vi "MOCVD_FrontPanel.vi"() -> ()   [LabVIEW 2011]
uses:
  low_level_proc/globals.vi
  editor_lib/Flow_Globals.vi
panel:
  out "Temp Actual":dbl caption="Actual (C)" format="%.2f"
  in  "Set":bool
  in  "Temp Setpoint":dbl caption="Setpoint (C)"
  in  "Heater":bool
  in  "Spinner":bool
  in  "Heater/Spinner Remote":bool caption="Remote"
  in  "Vac Remote":bool
  in  "Vac Exhaust":bool
  in  "Atm Exhaust":bool
  in  "Clear All Relays":bool
  in  "Stop":bool
  in  "?":enum32{"N2/H2", "Al", "Ga", "In", "P", "As"}(tab)
  in  "display N2 or H2":bool=TRUE
  in  "H2N2 Remote":bool caption="Remote"
  in  "N2 Target Flow":dbl caption="Target" min=0.0 max=1000.0
  in  "H2 Target Flow":dbl caption="Target" min=0.0 max=1000.0
  out "H2N2 Actual Flow":dbl caption="Actual"
  in  "N2 On":bool caption="On"
  in  "H2 On":bool caption="On"
  in  "Al Target Flow":dbl caption="Target" min=0.0 max=100.0 format="%.1f"
  out "Al Actual Flow":dbl caption="Actual" format="%.1f"
  in  "Al Remote":bool caption="Remote"
  in  "Al Active":bool caption="Active"
  in  "Al Bubbler In":bool caption="Bubbler In"
  in  "Al Run":bool caption="Run"
  out "Ga Actual Flow2":dbl caption="Actual" format="%.2f"
  out "Ga Actual Flow1":dbl caption="Actual" format="%.2f"
  out "Ga Actual Flow3":dbl caption="Actual"
  in  "Ga Target Flow 2":dbl caption="Target" min=0.0 max=10.0 format="%.2f"
  in  "Ga Target Flow 1":dbl caption="Target" min=0.0 max=1.0 format="%.2f"
  in  "Ga Active":bool caption="Active"
  in  "Ga Bubbler In":bool caption="Bubbler In"
  in  "Ga Run":bool caption="Run"
  in  "Ga H2 Dilute":bool caption="H2 Dilute"
  in  "Ga Remote":bool caption="Remote"
  in  "Ga Target Flow 3":dbl caption="Target" min=0.0 max=1000.0
  in  "In Target Flow":dbl caption="Target" min=0.0 max=100.0 format="%.1f"
  out "In Actual Flow":dbl caption="Actual" format="%.1f"
  in  "In Remote":bool caption="Remote"
  in  "In Active":bool caption="Active"
  in  "In Bubbler In":bool caption="Bubbler In"
  in  "In Run":bool caption="Run"
  in  "P_gas Target Flow":dbl caption="Target" min=0.0 max=1000.0 format="%.1f"
  out "P Actual Flow":dbl caption="Actual" format="%.1f"
  in  "P gas Remote":bool caption="Remote"
  in  "P gas Active":bool caption="Active"
  in  "P Gas In":bool caption="Gas In"
  in  "P gas Run":bool caption="Run"
  in  "P gas H2 Purge":bool caption="H2 Purge"
  in  "AsH3 gas Target Flow":dbl caption="Target" min=0.0 max=1000.0 format="%.2f"
  out "As Actual Flow":dbl caption="Actual" format="%.2f"
  in  "As gas Run":bool caption="Run"
  in  "As gas H2 Purge":bool caption="H2 Purge"
  in  "As gas Active":bool caption="Active"
  in  "As Gas In":bool caption="Gas In"
  in  "As gas Remote":bool caption="Remote"
  in  "6940B GPIB Address":string="23"
  # "Flow (0-10000 sccm)"
  # "N2"
  # "H2"
  # "N2"
  # "H2"
  # "Flow (0-100 sscm)"
  # "Flow 1 (0-10 sscm)"
  # "Flow 2 (0-10 sscm)"
  # "Flow 3 (0-1000 sscm)"
  # "Flow (0-100 sscm)"
  # "Flow (0-100 sscm)"
  # "Flow (0-10 sscm)"
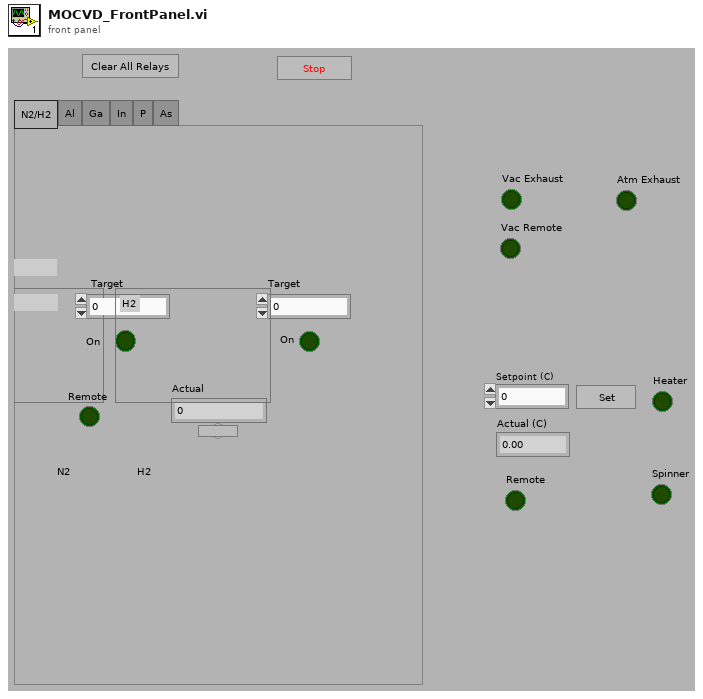
[diagram p1: front panel]
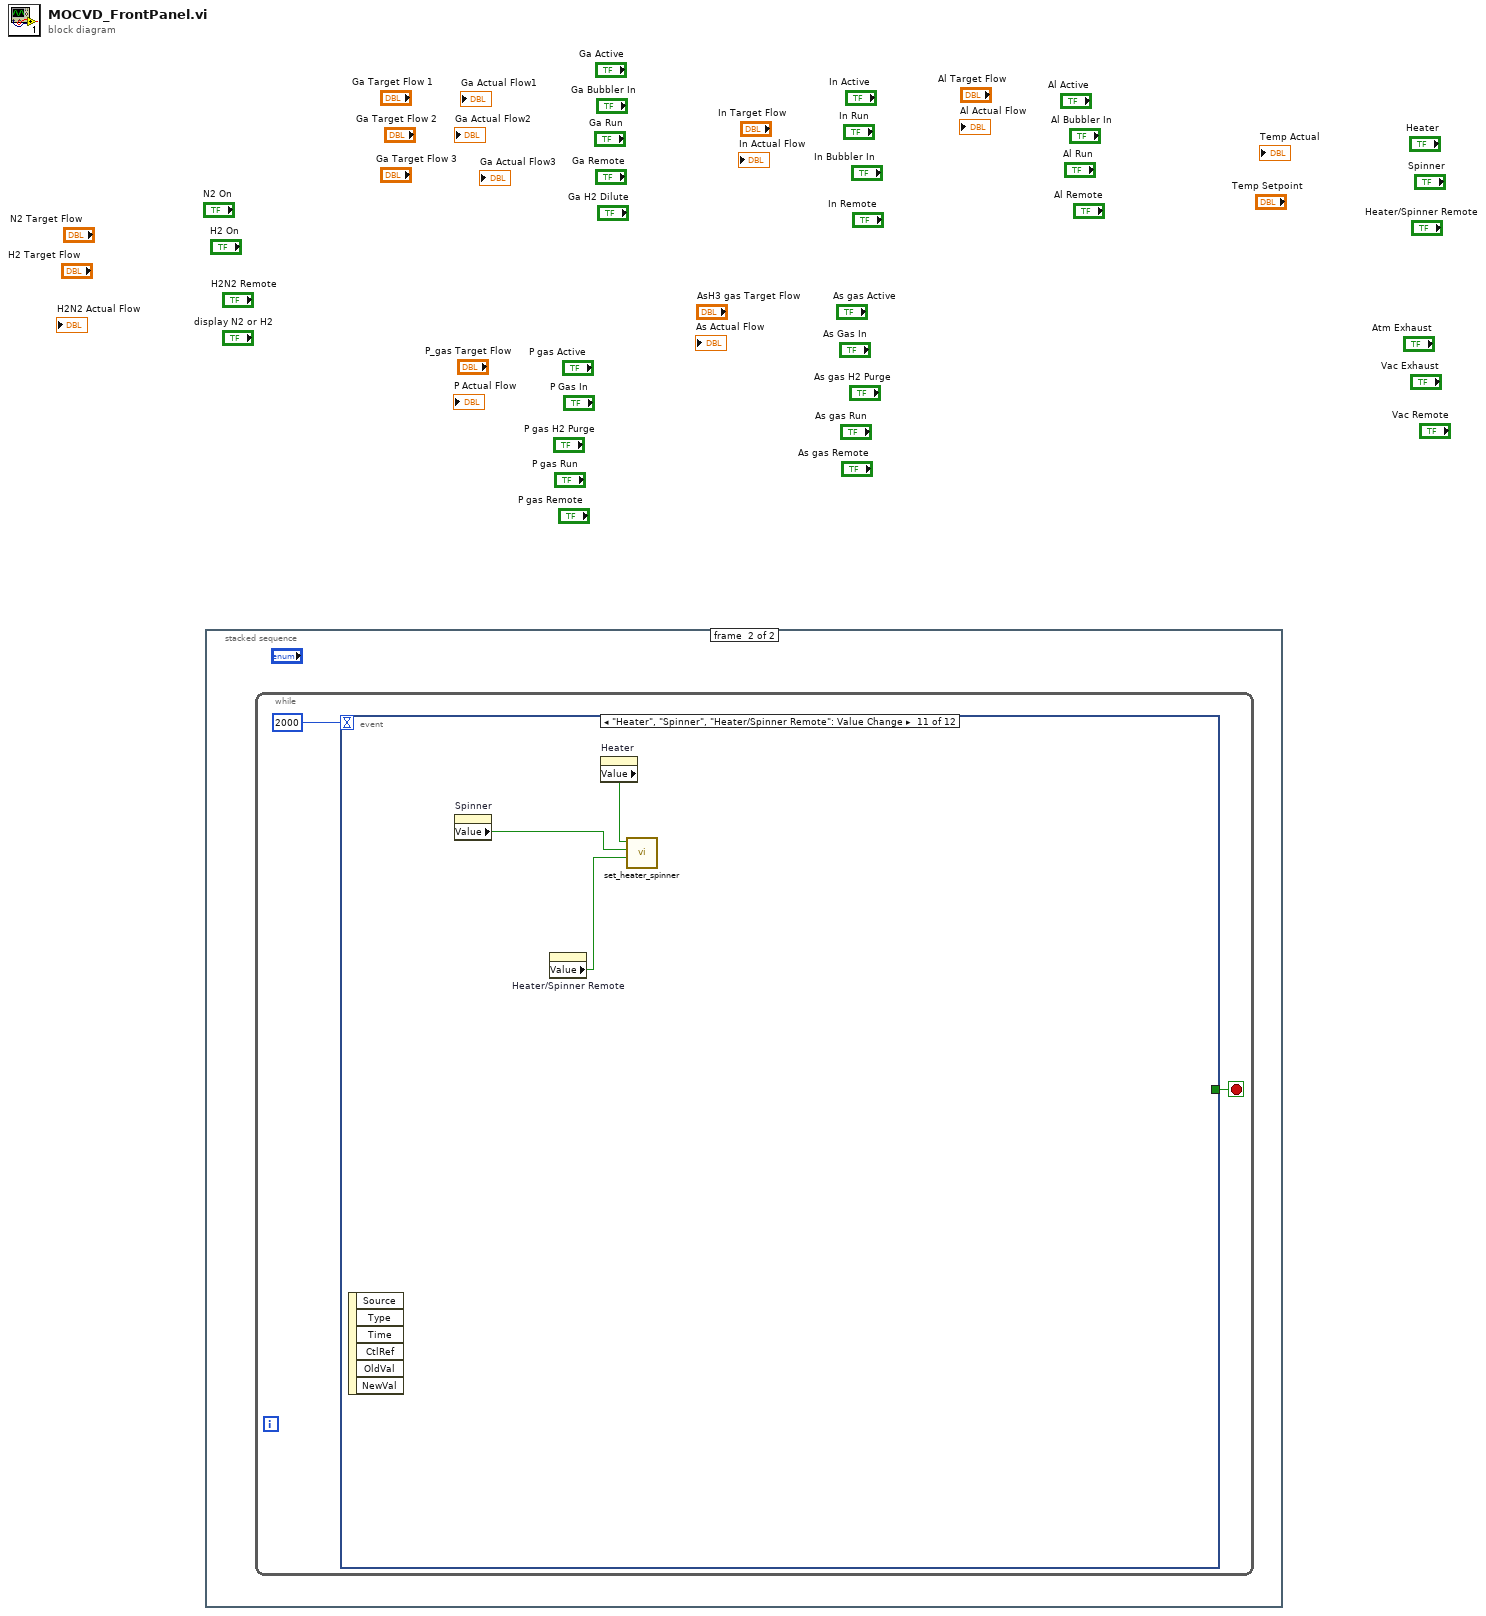
[diagram p0: block diagram]
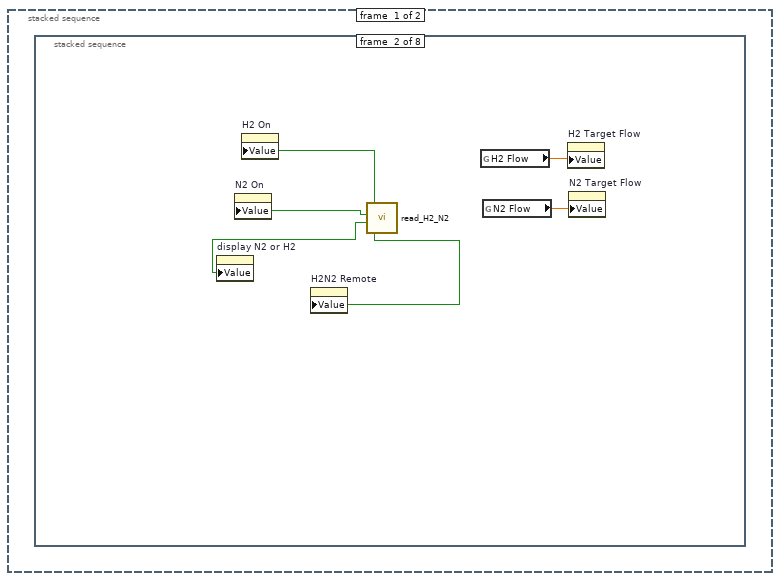
[diagram p2: hidden frame]
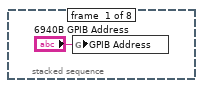
[diagram p3: hidden frame]
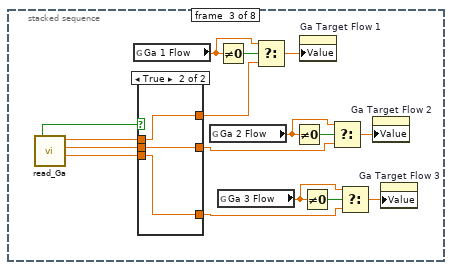
[diagram p4: hidden frame]
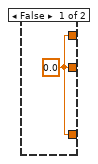
[diagram p5: hidden frame]
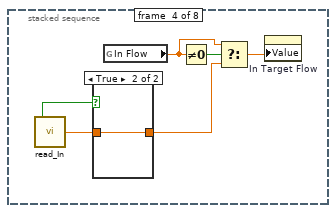
[diagram p6: hidden frame]
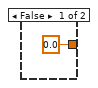
[diagram p7: hidden frame]
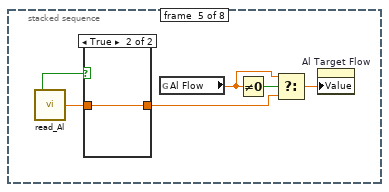
[diagram p8: hidden frame]
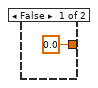
[diagram p9: hidden frame]
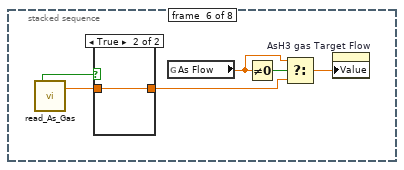
[diagram p10: hidden frame]
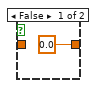
[diagram p11: hidden frame]
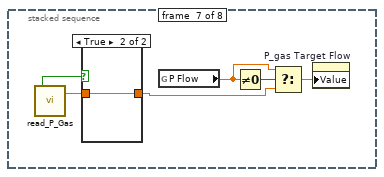
[diagram p12: hidden frame]
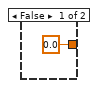
[diagram p13: hidden frame]
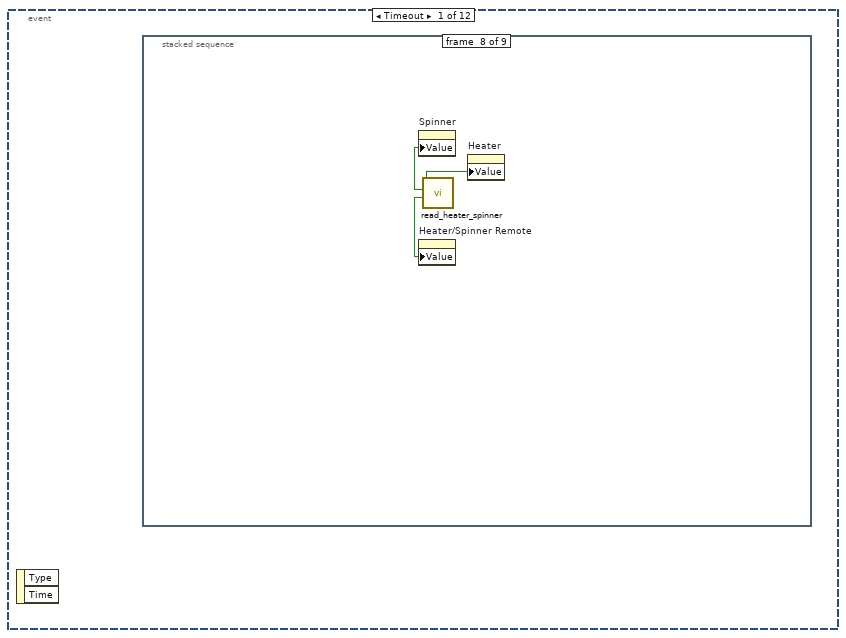
[diagram p15: hidden frame]
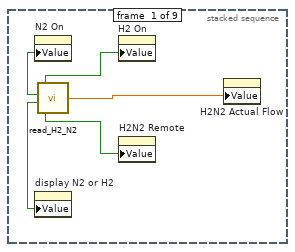
[diagram p16: hidden frame]
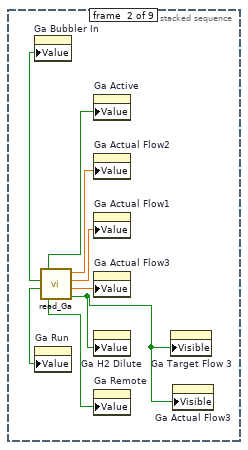
[diagram p17: hidden frame]
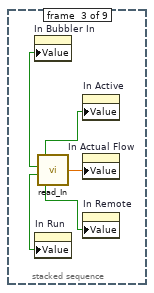
[diagram p18: hidden frame]
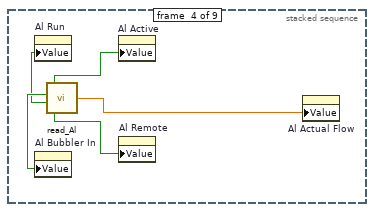
[diagram p19: hidden frame]
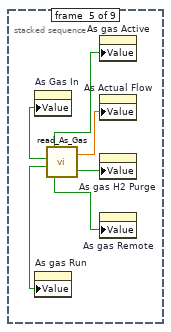
[diagram p20: hidden frame]
diagram:
  n1 = stacked-sequence {
    frame #0 {
      n2 = stacked-sequence {
        frame #0 {
          n3 = global write "globals.vi" "GPIB Address"("6940B GPIB Address") -> ()
        }
        frame #1 {
          n4 = call "read_H2_N2.vi"() -> ("H2N2 Remote"=w5:bool, "Display H2N2"=w4:bool, "N2 Active"=w7:bool, "H2 Active"=w6:bool)  [unwired: 1 out]
          n5 = property on="display N2 or H2" class="Bool (strict)"("Value"=w4) -> ()  [unwired: 2 in, 2 out]
          n6 = property on="N2 On" class="Bool (strict)"("Value"=w7) -> ()  [unwired: 2 in, 2 out]
          n7 = property on="H2 On" class="Bool (strict)"("Value"=w6) -> ()  [unwired: 2 in, 2 out]
          n8 = property on="H2N2 Remote" class="Bool (strict)"("Value"=w5) -> ()  [unwired: 2 in, 2 out]
          n9 = global read "Flow_Globals.vi" "H2 Flow"() -> (w3:dbl)
          n10 = global read "Flow_Globals.vi" "N2 Flow"() -> (w2:dbl)
          n11 = property on="H2 Target Flow" class="DigNum (strict)"("Value"=w3) -> ()  [unwired: 2 in, 2 out]
          n12 = property on="N2 Target Flow" class="DigNum (strict)"("Value"=w2) -> ()  [unwired: 2 in, 2 out]
        }
        frame #2 {
          n13 = call "read_Ga.vi"() -> ("GAMFC3"=w22:dbl, "GAMFC2"=w23:dbl, "GAMFC1"=w21:dbl, "Ga Active"=w20:bool)  [unwired: 4 out]
          n14 = global read "Flow_Globals.vi" "Ga 1 Flow"() -> (w18:dbl)
          n15 = case shown="True" w20 {
            tunnel: w23 -> [_ w26]
            tunnel: w22 -> [_ w25]
            tunnel: w21 -> [_ w27]
            tunnel: [w24 w27] -> w17
            tunnel: [w24 w26] -> w13
            tunnel: [w24 w25] -> w9
            frame False {
              w24 = 0.0 ("GAMFC2")
            }
            frame True {
            }
          }
          n16 = global read "Flow_Globals.vi" "Ga 2 Flow"() -> (w14:dbl)
          n17 = Not Equal To 0?(x=w18) -> (x != 0?=w19:bool)
          n18 = global read "Flow_Globals.vi" "Ga 3 Flow"() -> (w10:dbl)
          n19 = Select(t=w18, s=w19, f=w17) -> (s? t:f=w16:dbl)
          n20 = Not Equal To 0?(x=w14) -> (x != 0?=w15:bool)
          n21 = property on="Ga Target Flow 1" class="DigNum (strict)"("Value"=w16) -> ()  [unwired: 2 in, 2 out]
          n22 = Not Equal To 0?(x=w10) -> (x != 0?=w11:bool)
          n23 = Select(t=w14, s=w15, f=w13) -> (s? t:f=w12:dbl)
          n24 = Select(t=w10, s=w11, f=w9) -> (s? t:f=w8:dbl)
          n25 = property on="Ga Target Flow 2" class="DigNum (strict)"("Value"=w12) -> ()  [unwired: 2 in, 2 out]
          n26 = property on="Ga Target Flow 3" class="DigNum (strict)"("Value"=w8) -> ()  [unwired: 2 in, 2 out]
        }
        frame #3 {
          n27 = call "read_In.vi"() -> ("Actual In Flow Rate"=w32:dbl, "In Active"=w33:bool)  [unwired: 3 out]
          n28 = case shown="True" w33 {
            tunnel: [0.0 ("Actual In Flow Rate") w35] -> w29
            tunnel: w32 -> [_ w35]
            frame False {
            }
            frame True {
            }
          }
          n29 = global read "Flow_Globals.vi" "In Flow"() -> (w30:dbl)
          n30 = Not Equal To 0?(x=w30) -> (x != 0?=w31:bool)
          n31 = Select(t=w30, s=w31, f=w29) -> (s? t:f=w28:dbl)
          n32 = property on="In Target Flow" class="DigNum (strict)"("Value"=w28) -> ()  [unwired: 2 in, 2 out]
        }
        frame #4 {
          n33 = call "read_Al.vi"() -> ("Actual Al Flow Rate"=w41:dbl, "Al Active"=w40:bool)  [unwired: 3 out]
          n34 = case shown="True" w40 {
            tunnel: [0.0 ("Actual Al Flow Rate") w43] -> w37
            tunnel: w41 -> [_ w43]
            frame False {
            }
            frame True {
            }
          }
          n35 = global read "Flow_Globals.vi" "Al Flow"() -> (w38:dbl)
          n36 = Not Equal To 0?(x=w38) -> (x != 0?=w39:bool)
          n37 = Select(t=w38, s=w39, f=w37) -> (s? t:f=w36:dbl)
          n38 = property on="Al Target Flow" class="DigNum (strict)"("Value"=w36) -> ()  [unwired: 2 in, 2 out]
        }
        frame #5 {
          n39 = call "read_As_Gas.vi"() -> ("As Gas Actual Flow Rate"=w48:dbl, "As Gas Active"=w49:bool)  [unwired: 4 out]
          n40 = case shown="True" w49 {
            tunnel: w48 -> [_ w51]
            tunnel: [0.0 ("As Gas Actual Flow Rate") w51] -> w45
            frame False {
            }
            frame True {
            }
          }
          n41 = global read "Flow_Globals.vi" "As Flow"() -> (w46:dbl)
          n42 = Not Equal To 0?(x=w46) -> (x != 0?=w47:bool)
          n43 = Select(t=w46, s=w47, f=w45) -> (s? t:f=w44:dbl)
          n44 = property on="AsH3 gas Target Flow" class="DigNum (strict)"("Value"=w44) -> ()  [unwired: 2 in, 2 out]
        }
        frame #6 {
          n45 = call "read_P_Gas.vi"() -> ("P Gas Actual Flow Rate"=w56:dbl, "P Gas Active"=w57:bool)  [unwired: 4 out]
          n46 = case shown="True" w57 {
            tunnel: [0.0 ("P Gas Actual Flow Rate") w59] -> w53
            tunnel: w56 -> [_ w59]
            frame False {
            }
            frame True {
            }
          }
          n47 = global read "Flow_Globals.vi" "P Flow"() -> (w54:dbl)
          n48 = Not Equal To 0?(x=w54) -> (x != 0?=w55:bool)
          n49 = Select(t=w54, s=w55, f=w53) -> (s? t:f=w52:dbl)
          n50 = property on="P_gas Target Flow" class="DigNum (strict)"("Value"=w52) -> ()  [unwired: 2 in, 2 out]
        }
        frame #7 {
        }
      }
    }
    frame #1 {
      n51 = while {
        stop <- w61 stop-if-true
        n52 = event shown="[10] \"Heater\", \"Spinner\", \"Heater/Spinner Remote\": Value Change" {
          selector: _ -> [_ _ _ _ _ _ _ _ _ _ _ _]
          dyn-events: _ -> [_ _ _ _ _ _ _ _ _ _ _ _]
          timeout: 2000 -> [_ _ _ _ _ _ _ _ _ _ _ _]
          tunnel: [_ _ _ "Stop" _ _ _ _ _ _ _ _] -> w61
          event Timeout {
            n53 = event-data() -> ()  [unwired: 3 out]
            n54 = stacked-sequence {
              frame #0 {
                n55 = call "read_H2_N2.vi"() -> ("H2N2 Flow Rate"=w62:dbl, "H2N2 Remote"=w66:bool, "Display H2N2"=w65:bool, "N2 Active"=w64:bool, "H2 Active"=w63:bool)
                n56 = property on="N2 On" class="Bool (strict)"("Value"=w64) -> ()  [unwired: 2 in, 2 out]
                n57 = property on="display N2 or H2" class="Bool (strict)"("Value"=w65) -> ()  [unwired: 2 in, 2 out]
                n58 = property on="H2 On" class="Bool (strict)"("Value"=w63) -> ()  [unwired: 2 in, 2 out]
                n59 = property on="H2N2 Remote" class="Bool (strict)"("Value"=w66) -> ()  [unwired: 2 in, 2 out]
                n60 = property on="H2N2 Actual Flow" class="DigNum (strict)"("Value"=w62) -> ()  [unwired: 2 in, 2 out]
              }
              frame #1 {
                n61 = call "read_Ga.vi"() -> ("H2 Dilute"=w67:bool, "GAMFC3"=w68:dbl, "GAMFC2"=w70:dbl, "GAMFC1"=w69:dbl, "Ga Remote"=w73:bool, "Ga Run"=w74:bool, "Ga Bubbler"=w71:bool, "Ga Active"=w72:bool)
                n62 = property on="Ga Bubbler In" class="Bool (strict)"("Value"=w71) -> ()  [unwired: 2 in, 2 out]
                n63 = property on="Ga Run" class="Bool (strict)"("Value"=w74) -> ()  [unwired: 2 in, 2 out]
                n64 = property on="Ga Active" class="Bool (strict)"("Value"=w72) -> ()  [unwired: 2 in, 2 out]
                n65 = property on="Ga Actual Flow2" class="DigNum (strict)"("Value"=w69) -> ()  [unwired: 2 in, 2 out]
                n66 = property on="Ga Actual Flow1" class="DigNum (strict)"("Value"=w70) -> ()  [unwired: 2 in, 2 out]
                n67 = property on="Ga Actual Flow3" class="DigNum (strict)"("Value"=w68) -> ()  [unwired: 2 in, 2 out]
                n68 = property on="Ga H2 Dilute" class="Bool (strict)"("Value"=w67) -> ()  [unwired: 2 in, 2 out]
                n69 = property on="Ga Remote" class="Bool (strict)"("Value"=w73) -> ()  [unwired: 2 in, 2 out]
                n70 = property on="Ga Target Flow 3" class="DigNum (strict)"("Visible"=w67) -> ()  [unwired: 2 in, 2 out]
                n71 = property on="Ga Actual Flow3" class="DigNum (strict)"("Visible"=w67) -> ()  [unwired: 2 in, 2 out]
              }
              frame #2 {
                n72 = call "read_In.vi"() -> ("Actual In Flow Rate"=w75:dbl, "In Remote"=w77:bool, "In Run"=w76:bool, "In Bubbler"=w78:bool, "In Active"=w79:bool)
                n73 = property on="In Bubbler In" class="Bool (strict)"("Value"=w78) -> ()  [unwired: 2 in, 2 out]
                n74 = property on="In Run" class="Bool (strict)"("Value"=w76) -> ()  [unwired: 2 in, 2 out]
                n75 = property on="In Active" class="Bool (strict)"("Value"=w79) -> ()  [unwired: 2 in, 2 out]
                n76 = property on="In Actual Flow" class="DigNum (strict)"("Value"=w75) -> ()  [unwired: 2 in, 2 out]
                n77 = property on="In Remote" class="Bool (strict)"("Value"=w77) -> ()  [unwired: 2 in, 2 out]
              }
              frame #3 {
                n78 = call "read_Al.vi"() -> ("Actual Al Flow Rate"=w80:dbl, "Al Remote"=w81:bool, "Al Run"=w82:bool, "Al Bubbler"=w83:bool, "Al Active"=w84:bool)
                n79 = property on="Al Run" class="Bool (strict)"("Value"=w82) -> ()  [unwired: 2 in, 2 out]
                n80 = property on="Al Bubbler In" class="Bool (strict)"("Value"=w83) -> ()  [unwired: 2 in, 2 out]
                n81 = property on="Al Active" class="Bool (strict)"("Value"=w84) -> ()  [unwired: 2 in, 2 out]
                n82 = property on="Al Remote" class="Bool (strict)"("Value"=w81) -> ()  [unwired: 2 in, 2 out]
                n83 = property on="Al Actual Flow" class="DigNum (strict)"("Value"=w80) -> ()  [unwired: 2 in, 2 out]
              }
              frame #4 {
                n84 = call "read_As_Gas.vi"() -> ("As Gas H2 In"=w86:bool, "As Gas Actual Flow Rate"=w85:dbl, "As Gas Remote"=w90:bool, "As Gas Run"=w89:bool, "As Gas In"=w88:bool, "As Gas Active"=w87:bool)
                n85 = property on="As Gas In" class="Bool (strict)"("Value"=w88) -> ()  [unwired: 2 in, 2 out]
                n86 = property on="As gas Run" class="Bool (strict)"("Value"=w89) -> ()  [unwired: 2 in, 2 out]
                n87 = property on="As gas Active" class="Bool (strict)"("Value"=w87) -> ()  [unwired: 2 in, 2 out]
                n88 = property on="As Actual Flow" class="DigNum (strict)"("Value"=w85) -> ()  [unwired: 2 in, 2 out]
                n89 = property on="As gas H2 Purge" class="Bool (strict)"("Value"=w86) -> ()  [unwired: 2 in, 2 out]
                n90 = property on="As gas Remote" class="Bool (strict)"("Value"=w90) -> ()  [unwired: 2 in, 2 out]
              }
              frame #5 {
                n91 = call "read_P_Gas.vi"() -> ("P Gas H2 In"=w92:bool, "P Gas Actual Flow Rate"=w91:dbl, "P Gas Remote"=w96:bool, "P Gas Run"=w95:bool, "P Gas In"=w94:bool, "P Gas Active"=w93:bool)
                n92 = property on="P Gas In" class="Bool (strict)"("Value"=w94) -> ()  [unwired: 2 in, 2 out]
                n93 = property on="P gas Run" class="Bool (strict)"("Value"=w95) -> ()  [unwired: 2 in, 2 out]
                n94 = property on="P gas Active" class="Bool (strict)"("Value"=w93) -> ()  [unwired: 2 in, 2 out]
                n95 = property on="P Actual Flow" class="DigNum (strict)"("Value"=w91) -> ()  [unwired: 2 in, 2 out]
                n96 = property on="P gas H2 Purge" class="Bool (strict)"("Value"=w92) -> ()  [unwired: 2 in, 2 out]
                n97 = property on="P gas Remote" class="Bool (strict)"("Value"=w96) -> ()  [unwired: 2 in, 2 out]
              }
              frame #6 {
                n98 = call "read_vacuum.vi"() -> ("Vac Remote"=w99:bool, "Atm Exhaust"=w98:bool, "Vac Exhaust"=w97:bool)
                n99 = property on="Vac Exhaust" class="Bool (strict)"("Value"=w97) -> ()  [unwired: 2 in, 2 out]
                n100 = property on="Atm Exhaust" class="Bool (strict)"("Value"=w98) -> ()  [unwired: 2 in, 2 out]
                n101 = property on="Vac Remote" class="Bool (strict)"("Value"=w99) -> ()  [unwired: 2 in, 2 out]
              }
              frame #7 {
                n102 = call "read_heater_spinner.vi"() -> ("Heater/Spinner Remote"=w102:bool, "Spinner"=w101:bool, "Heater"=w100:bool)  [unwired: 7 out]
                n103 = property on="Spinner" class="Bool (strict)"("Value"=w101) -> ()  [unwired: 2 in, 2 out]
                n104 = property on="Heater/Spinner Remote" class="Bool (strict)"("Value"=w102) -> ()  [unwired: 2 in, 2 out]
                n105 = property on="Heater" class="Bool (strict)"("Value"=w100) -> ()  [unwired: 2 in, 2 out]
              }
              frame #8 {
                n106 = call "read_temp.vi"() -> ("Temperature (C)"=w103:dbl)  [unwired: 1 out]
                n107 = property on="Temp Actual" class="DigNum (strict)"("Value"=w103) -> ()  [unwired: 2 in, 2 out]
              }
            }
          }
          event "Set": Value Change {
            n108 = event-data() -> ()  [unwired: 6 out]
            n109 = property on="Temp Setpoint" class="DigNum (strict)"() -> ("Value"=w104:dbl)  [unwired: 2 in, 2 out]
            n110 = call "write_temp.vi"("Temperature (C)"=w104) -> ()  [unwired: 1 out]
          }
          event "Clear All Relays": Mouse Down {
            n111 = event-data() -> ()  [unwired: 8 out]
            n112 = flat-sequence {
              frame #0 {
                n113 = call "clear_all_relays.vi"() -> ()  [unwired: 2 out]
              }
              frame #1 {
                n114 = property on="Clear All Relays" class="Bool (strict)"("Value"=FALSE ("Clear All Relays")) -> ()  [unwired: 2 in, 2 out]
              }
            }
          }
          event "Stop": Value Change {
            n115 = event-data() -> ()  [unwired: 7 out]
          }
          event "H2N2 Remote", "display N2 or H2", "N2 On", "H2 On", "N2 Target Flow", "H2 Target Flow": Value Change {
            n116 = event-data() -> ()  [unwired: 7 out]
            n117 = property on="H2 On" class="Bool (strict)"() -> ("Value"=w111:bool)  [unwired: 2 in, 2 out]
            n118 = property on="N2 Target Flow" class="DigNum (strict)"() -> ("Value"=w108:dbl)  [unwired: 2 in, 2 out]
            n119 = property on="H2N2 Remote" class="Bool (strict)"() -> ("Value"=w109:bool)  [unwired: 2 in, 2 out]
            n120 = property on="H2 Target Flow" class="DigNum (strict)"() -> ("Value"=w107:dbl)  [unwired: 2 in, 2 out]
            n121 = property on="N2 On" class="Bool (strict)"() -> ("Value"=w112:bool)  [unwired: 2 in, 2 out]
            n122 = property on="display N2 or H2" class="Bool (strict)"() -> ("Value"=w110:bool)  [unwired: 2 in, 2 out]
            n123 = call "set_N2.vi"("Manifold N2 Flow"=w108, "Display H2 or N2"=w110, "N2 Active"=w112, "H2N2 Remote"=w109) -> ()  [unwired: 2 out]
            n124 = call "set_H2.vi"("Manifold H2 Flow"=w107, "Display H2 or N2"=w110, "H2 Active"=w111, "H2N2 Remote"=w109) -> ()  [unwired: 2 in]
          }
          event "In Remote", "In Active", "In Bubbler In", "In Run", "In Target Flow": Value Change {
            n125 = event-data() -> ()  [unwired: 7 out]
            n126 = property on="In Target Flow" class="DigNum (strict)"() -> ("Value"=w117:dbl)  [unwired: 2 in, 2 out]
            n127 = property on="In Bubbler In" class="Bool (strict)"() -> ("Value"=w115:bool)  [unwired: 2 in, 2 out]
            n128 = property on="In Run" class="Bool (strict)"() -> ("Value"=w114:bool)  [unwired: 2 in, 2 out]
            n129 = property on="In Active" class="Bool (strict)"() -> ("Value"=w116:bool)  [unwired: 2 in, 2 out]
            n130 = property on="In Remote" class="Bool (strict)"() -> ("Value"=w113:bool)  [unwired: 2 in, 2 out]
            n131 = call "set_In.vi"("Indium Flow"=w117, "In Remote"=w113, "In Run"=w114, "In Bubbler"=w115, "In Active"=w116) -> ()  [unwired: 5 out]
          }
          event "Al Remote", "Al Active", "Al Bubbler In", "Al Run", "Al Target Flow": Value Change {
            n132 = event-data() -> ()  [unwired: 7 out]
            n133 = property on="Al Target Flow" class="DigNum (strict)"() -> ("Value"=w122:dbl)  [unwired: 2 in, 2 out]
            n134 = property on="Al Bubbler In" class="Bool (strict)"() -> ("Value"=w120:bool)  [unwired: 2 in, 2 out]
            n135 = property on="Al Active" class="Bool (strict)"() -> ("Value"=w121:bool)  [unwired: 2 in, 2 out]
            n136 = property on="Al Run" class="Bool (strict)"() -> ("Value"=w119:bool)  [unwired: 2 in, 2 out]
            n137 = property on="Al Remote" class="Bool (strict)"() -> ("Value"=w118:bool)  [unwired: 2 in, 2 out]
            n138 = call "set_Al.vi"("Aluminum Flow"=w122, "Al Remote"=w118, "Al Run"=w119, "Al Bubbler"=w120, "Al Active"=w121) -> ()  [unwired: 5 out]
          }
          event "P gas Remote", "P gas Active", "P Gas In", "P gas Run", "P gas H2 Purge", "P_gas Target Flow": Value Change {
            n139 = event-data() -> ()  [unwired: 7 out]
            n140 = property on="P_gas Target Flow" class="DigNum (strict)"() -> ("Value"=w128:dbl)  [unwired: 2 in, 2 out]
            n141 = property on="P gas Active" class="Bool (strict)"() -> ("Value"=w127:bool)  [unwired: 2 in, 2 out]
            n142 = property on="P Gas In" class="Bool (strict)"() -> ("Value"=w126:bool)  [unwired: 2 in, 2 out]
            n143 = property on="P gas H2 Purge" class="Bool (strict)"() -> ("Value"=w125:bool)  [unwired: 2 in, 2 out]
            n144 = property on="P gas Run" class="Bool (strict)"() -> ("Value"=w124:bool)  [unwired: 2 in, 2 out]
            n145 = property on="P gas Remote" class="Bool (strict)"() -> ("Value"=w123:bool)  [unwired: 2 in, 2 out]
            n146 = call "set_P_gas.vi"("P_Gas Active"=w127, "P_Gas Flow"=w128, "P_Gas In"=w126, "P_Gas H2 In"=w125, "P_Gas Run"=w124, "P_Gas Remote"=w123) -> ()  [unwired: 10 out]
          }
          event "As gas Remote", "As gas Run", "As gas H2 Purge", "As Gas In", "As gas Active", "AsH3 gas Target Flow": Value Change {
            n147 = event-data() -> ()  [unwired: 7 out]
            n148 = property on="AsH3 gas Target Flow" class="DigNum (strict)"() -> ("Value"=w134:dbl)  [unwired: 2 in, 2 out]
            n149 = property on="As gas Active" class="Bool (strict)"() -> ("Value"=w133:bool)  [unwired: 2 in, 2 out]
            n150 = property on="As Gas In" class="Bool (strict)"() -> ("Value"=w132:bool)  [unwired: 2 in, 2 out]
            n151 = property on="As gas H2 Purge" class="Bool (strict)"() -> ("Value"=w131:bool)  [unwired: 2 in, 2 out]
            n152 = property on="As gas Run" class="Bool (strict)"() -> ("Value"=w130:bool)  [unwired: 2 in, 2 out]
            n153 = property on="As gas Remote" class="Bool (strict)"() -> ("Value"=w129:bool)  [unwired: 2 in, 2 out]
            n154 = call "set_As_gas.vi"("As_Gas Active"=w133, "As_Gas Flow"=w134, "As_Gas In"=w132, "As_Gas H2"=w131, "As_Gas Run"=w130, "As_Gas Remote"=w129) -> ()  [unwired: 10 out]
          }
          event "Ga Active", "Ga Bubbler In", "Ga Run", "Ga Target Flow 1", "Ga Target Flow 2", "Ga Target Flow 3", "Ga Remote", "Ga H2 Dilute": Value Change {
            n155 = event-data() -> ()  [unwired: 6 out]
            n156 = property on="Ga Bubbler In" class="Bool (strict)"() -> ("Value"=w139:bool)  [unwired: 2 in, 2 out]
            n157 = property on="Ga Target Flow 1" class="DigNum (strict)"() -> ("Value"=w142:dbl)  [unwired: 2 in, 2 out]
            n158 = property on="Ga Target Flow 2" class="DigNum (strict)"() -> ("Value"=w141:dbl)  [unwired: 2 in, 2 out]
            n159 = property on="Ga Target Flow 3" class="DigNum (strict)"() -> ("Value"=w140:dbl)  [unwired: 2 in, 2 out]
            n160 = property on="Ga Active" class="Bool (strict)"() -> ("Value"=w138:bool)  [unwired: 2 in, 2 out]
            n161 = property on="Ga Run" class="Bool (strict)"() -> ("Value"=w136:bool)  [unwired: 2 in, 2 out]
            n162 = property on="Ga Remote" class="Bool (strict)"() -> ("Value"=w137:bool)  [unwired: 2 in, 2 out]
            n163 = property on="Ga H2 Dilute" class="Bool (strict)"() -> ("Value"=w135:bool)  [unwired: 2 in, 2 out]
            n164 = call "set_Ga.vi"("Ga Active"=w138, "Ga Flow 3"=w140, "Ga Flow 2"=w141, "Ga Flow 1"=w142, "Ga Bubbler"=w139, "Ga H2 Dilute"=w135, "Ga Run"=w136, "Ga Remote"=w137) -> ()  [unwired: 8 out]
            n165 = property on="Ga Target Flow 3" class="DigNum (strict)"("Visible"=w135) -> ()  [unwired: 2 in, 2 out]
            n166 = property on="Ga Actual Flow3" class="DigNum (strict)"("Visible"=w135) -> ()  [unwired: 2 in, 2 out]
          }
          event "Heater", "Spinner", "Heater/Spinner Remote": Value Change {
            n167 = event-data() -> ()  [unwired: 7 out]
            n168 = property on="Spinner" class="Bool (strict)"() -> ("Value"=w143:bool)  [unwired: 2 in, 2 out]
            n169 = property on="Heater/Spinner Remote" class="Bool (strict)"() -> ("Value"=w145:bool)  [unwired: 2 in, 2 out]
            n170 = property on="Heater" class="Bool (strict)"() -> ("Value"=w144:bool)  [unwired: 2 in, 2 out]
            n171 = call "set_heater_spinner.vi"("Heater/Spinner Remote"=w145, "Spinner"=w143, "Heater"=w144) -> ()  [unwired: 7 out]
          }
          event "Vac Remote", "Vac Exhaust", "Atm Exhaust": Value Change {
            n172 = event-data() -> ()  [unwired: 7 out]
            n173 = property on="Vac Remote" class="Bool (strict)"() -> ("Value"=w148:bool)  [unwired: 2 in, 2 out]
            n174 = property on="Vac Exhaust" class="Bool (strict)"() -> ("Value"=w147:bool)  [unwired: 2 in, 2 out]
            n175 = property on="Atm Exhaust" class="Bool (strict)"() -> ("Value"=w146:bool)  [unwired: 2 in, 2 out]
            n176 = call "set_vacuum.vi"("Vac Remote"=w148, "Atm Exhaust"=w146, "Vac Exhaust"=w147) -> ()
          }
        }
      }
    }
  }
